vi "ScopeCHConfig.vi"(6 "enable":bool=TRUE, 8 "error in (no error)":errorcluster caption="错误输入（无错误）", 9 "range(V)":dbl=5.0, 10 "CH":i32, 11 "handle":u64) -> (0 "error out":errorcluster caption="错误输出", 2 "function return":i32, 3 "handle out":u64)   [LabVIEW 2018]
doc: "Select Scope Channel by CH ,then set range and whiter enable this channel"
uses:
  InstrumentsPlayground.lvlib
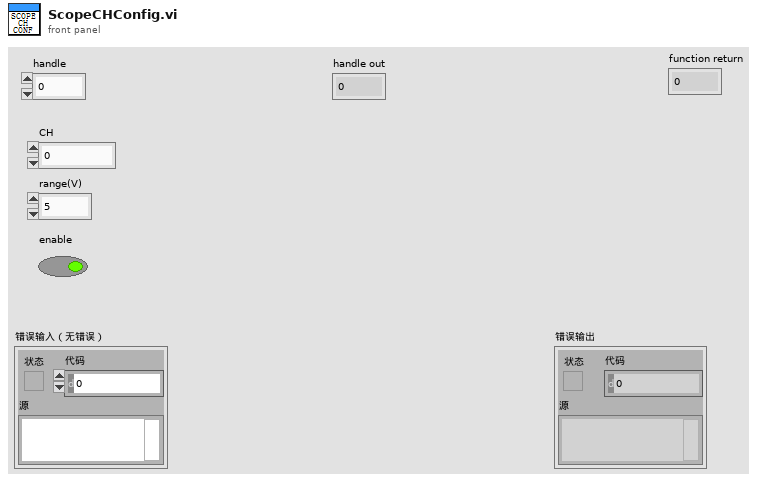
[diagram p1: front panel]
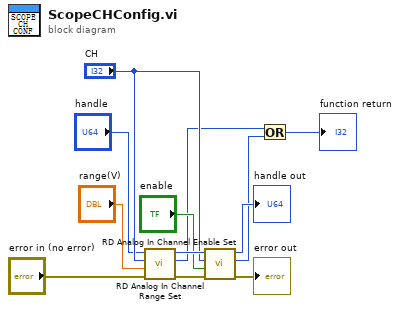
[diagram p0: block diagram]
diagram:
  n1 = call "RD Analog In Channel Range Set.vi"("error in (no error)"="error in (no error)", "range"="range(V)", "channel"="CH", "handle"="handle") -> ("error out"=w11:errorcluster, "function return"=w1:i32, "handle out"=w12:u64)  [unwired: 5 in]
  n2 = call "RD Analog In Channel Enable Set.vi"("error in (no error)"=w11, "enable"="enable", "channel"="CH", "handle"=w12) -> ("error out"=→"error out":errorcluster, "function return"=w3:i32, "handle out"=→"handle out":u64)  [unwired: 5 in]
  n3 = Or(x=w1, y=w3) -> (x .or. y?=→"function return":i32)
